vi "test_F9P_fgv-ver.vi"() -> ()   [LabVIEW 2019] (continued)
27,182,,07,09,201,18,1*72\r\n$GBGSV,4,2,13,08,65,355,33,09,07,194,,10,16,222,18,11,38,142,27,1*7C\r\n$GBGSV,4,3,13,13,50,314,20,14,77,038,37,28,58,310,28,33,72,237,41,1*73\r\n$GBGSV,4,4,13,34,13,141,,1*45\r\n$GBGSV,4,1,13,04,35,133,,05,09,257,,06,27,182,,07,09,201,,3*79\r\n$GBGSV,4,2,13,08,65,355,33,09,07,194,,10,16,222,19,11,38,142,26,3*7E\r\n$GBGSV,4,3,13,13,50,314,,14,77,038,38,28,58,310,,33,72,237,,3*73\r\n$GBGSV,4,4,13,34,13,141,,3*47\r\n$GNGLL,3723.61077,N,12656.95320,E,064222.00,A,A*7E\r\n$GNRMC,064223.00,A,3723.61113,N,12656.95407,E,2.484,70.88,250720,,,A,V*3C\r\n$GNVTG,70.88,T,,M,2.484,N,4.600,K,A*1C\r\n$GNGGA,064223.00,3723.61113,N,12656.95407,E,1,12,0.73,46.5,M,18.5,M,,*77\r\n$GNGSA,A,3,17,19,06,05,02,12,09,,,,,,1.16,0.73,0.90,1*0F\r\n$GNGSA,A,3,85,70,71,72,,,,,,,,,1.16,0.73,0.90,2*00\r\n$GNGSA,A,3,36,19,11,04,09,12,,,,,,,1.16,0.73,0.90,3*0B\r\n$GNGSA,A,3,28,14,13,11,33,08,10,,,,,,1.16,0.73,0.90,4*0B\r\n$GPGSV,4,1,13,02,65,334,31,04,08,037,26,05,48,261,35,06,58,076,40,1*6C\r\n$GPGSV,4,2,13,07,06,105,,09,38,057,43,12,18,263,24,13,08,191,,1*6A\r\n$GPGSV,4,3,13,17,19,158,25,19,37,161,34,25,11,294,18,29,07,323,,1*66\r\n$GPGSV,4,4,13,30,01,134,,1*52\r\n$GPGSV,4,1,13,02,65,334,,04,08,037,20,05,48,261,26,06,58,076,31,6*6B\r\n$GPGSV,4,2,13,07,06,105,,09,38,057,40,12,18,263,14,13,08,191,,6*6D\r\n$GPGSV,4,3,13,17,19,158,19,19,37,161,,25,11,294,,29,07,323,,6*60\r\n$GPGSV,4,4,13,30,01,134,,6*55\r\n$GLGSV,2,1,06,70,55,030,38,71,68,223,41,72,17,216,26,84,09,133,10,1*7B\r\n$GLGSV,2,2,06,85,63,111,34,86,51,337,,1*7D\r\n$GLGSV,2,1,06,70,55,030,,71,68,223,28,72,17,216,20,84,09,133,10,3*7B\r\n$GLGSV,2,2,06,85,63,111,25,86,51,337,,3*7F\r\n$GAGSV,3,1,09,02,04,287,10,04,68,085,41,09,44,196,30,11,78,037,38,7*74\r\n$GAGSV,3,2,09,12,32,114,28,18,55,286,40,19,17,042,27,25,01,241,,7*7A\r\n$GAGSV,3,3,09,36,34,314,23,7*4F\r\n$GAGSV,3,1,09,02,04,287,,04,68,085,31,09,44,196,28,11,78,037,31,2*77\r\n$GAGSV,3,2,09,12,32,114,25,18,55,286,43,19,17,042,25,25,01,241,,2*73\r\n$GAGSV,3,3,09,36,34,314,19,2*43\r\n$GBGSV,4,1,13,04,35,133,,05,09,257,,06,27,182,,07,09,201,19,1*73\r\n$GBGSV,4,2,13,08,65,355,39,09,07,194,,10,16,222,17,11,38,142,26,1*78\r\n$GBGSV,4,3,13,13,50,314,20,14,77,038,38,28,58,310,28,33,72,237,42,1*7F\r\n$GBGSV,4,4,13,34,13,141,,1*45\r\n$GBGSV,4,1,13,04,35,133,,05,09,257,,06,27,182,,07,09,201,,3*79\r\n$GBGSV,4,2,13,08,65,355,37,09,07,194,,10,16,222,20,11,38,142,30,3*77\r\n$GBGSV,4,3,13,13,50,314,,14,77,038,40,28,58,310,,33,72,237,,3*7C\r\n$GBGSV,4,4,13,34,13,141,,3*47\r\n$GNGLL,3723.61113,N,12656.95407,E,064223.00,A,A*7E\r\n$GNRMC,064224.00,A,3723.61154,N,12656.95489,E,2.441,65.71,250720,,,A,V*35\r\n$GNVTG,65.71,T,,M,2.441,N,4.520,K,A*16\r\n$GNGGA,064224.00,3723.61154,N,12656.95489,E,1,12,0.73,46.1,M,18.5,M,,*71\r\n$GNGSA,A,3,17,19,06,05,02,12,09,,,,,,1.16,0.73,0.90,1*0F\r\n$GNGSA,A,3,85,70,71,72,,,,,,,,,1.16,0.73,0.90,2*00\r\n$GNGSA,A,3,36,19,11,04,09,12,,,,,,,1.16,0.73,0.90,3*0B\r\n$GNGSA,A,3,28,14,13,11,33,08,10,,,,,,1.16,0.73,0.90,4*0B\r\n$GPGSV,4,1,13,02,65,334,26,04,08,037,32,05,48,261,35,06,58,076,42,1*6D\r\n$GPGSV,4,2,13,07,06,105,,09,38,057,44,12,18,263,23,13,08,191,,1*6A\r\n$GPGSV,4,3,13,17,19,158,26,19,37,161,31,25,11,294,18,29,07,323,,1*60\r\n$GPGSV,4,4,13,30,01,134,,1*52\r\n$GPGSV,4,1,13,02,65,334,,04,08,037,20,05,48,261,26,06,58,076,32,6*68\r\n$GPGSV,4,2,13,07,06,105,,09,38,057,39,12,18,263,15,13,08,191,,6*62\r\n$GPGSV,4,3,13,17,19,158,21,19,37,161,,25,11,294,,29,07,323,,6*6B\r\n$GPGSV,4,4,13,30,01,134,,6*55\r\n$GLGSV,2,1,06,70,55,030,36,71,68,223,42,72,17,216,35,84,09,133,10,1*74\r\n$GLGSV,2,2,06,85,63,111,25,86,51,337,,1*7D\r\n$GLGSV,2,1,06,70,55,030,,71,68,223,28,72,17,216,21,84,09,133,10,3*7A\r\n$GLGSV,2,2,06,85,63,111,24,86,51,337,,3*7E\r\n$GAGSV,3,1,09,02,04,287,09,04,68,085,37,09,44,196,29,11,78,037,36,7*7B\r\n$GAGSV,3,2,09,12,32,114,32,18,55,286,35,19,17,042,28,25,01,241,,7*7C\r\n$GAGSV,3,3,09,36,34,314,24,7*48\r\n$GAGSV,3,1,09,02,04,287,,04,68,085,35,09,44,196,27,11,78,037,32,2*7F\r\n$GAGSV,3,2,09,12,32,114,25,18,55,286,43,19,17,042,31,25,01,241,,2*76\r\n$GAGSV,3,3,09,36,34,314,19,2*43\r\n$GBGSV,4,1,13,04,35,133,,05,09,257,,06,27,182,,07,09,201,20,1*79\r\n$GBGSV,4,2,13,08,65,355,40,09,07,194,,10,16,222,16,11,38,142,27,1*76\r\n$GBGSV,4,3,13,13,50,314,19,14,77,038,42,28,58,310,26,33,72,237,33,1*70\r\n$GBGSV,4,4,13,34,13,141,,1*45\r\n$GBGSV,4,1,13,04,35,133,,05,09,257,,06,27,182,,07,09,201,,3*79\r\n$GBGSV,4,2,13,08,65,355,36,09,07,194,,10,16,222,20,11,38,142,29,3*7E\r\n$GBGSV,4,3,13,13,50,314,,14,77,038,37,28,58,310,,33,72,237,,3*7C\r\n$GBGSV,4,4,13,34,13,141,,3*47\r\n$GNGLL,3723.61154,N,12656.95489,E,064224.00,A,A*7C\r\n$GNRMC,064225.00,A,3723.61204,N,12656.95562,E,2.487,60.20,250720,,,A,V*3D\r\n$GNVTG,60.20,T,,M,2.487,N,4.606,K,A*1A\r\n$GNGGA,064225.00,3723.61204,N,12656.95562,E,1,12,0.76,45.7,M,18.5,M,,*72\r\n$GNGSA,A,3,17,19,06,05,02,12,09,,,,,,1.18,0.76,0.90,1*04\r\n$GNGSA,A,3,85,70,71,72,,,,,,,,,1.18,0.76,0.90,2*0B\r\n$GNGSA,A,3,36,19,11,04,09,12,,,,,,,1.18,0.76,0.90,3*00\r\n$GNGSA,A,3,28,14,13,11,33,08,10,,,,,,1.18,0.76,0.90,4*00\r\n$GPGSV,4,1,13,02,65,334,36,04,08,037,28,05,48,261,32,06,58,076,36,1*63\r\n$GPGSV,4,2,13,07,06,105,,09,38,057,43,12,18,263,25,13,08,191,,1*6B\r\n$GPGSV,4,3,13,17,19,158,26,19,37,161,26,25,11,294,17,29,07,323,,1*69\r\n$GPGSV,4,4,13,30,01,134,,1*52\r\n$GPGSV,4,1,13,02,65,334,,04,08,037,24,05,48,261,32,06,58,076,32,6*69\r\n$GPGSV,4,2,13,07,06,105,,09,38,057,39,12,18,263,15,13,08,191,,6*62\r\n$GPGSV,4,3,13,17,19,158,20,19,37,161,,25,11,294,,29,07,323,,6*6A\r\n$GPGSV,4,4,13,30,01,134,,6*55\r\n$GLGSV,2,1,06,70,55,030,40,71,68,223,37,72,17,216,30,84,09,133,07,1*74\r\n$GLGSV,2,2,06,85,63,111,34,86,51,337,,1*7D\r\n$GLGSV,2,1,06,70,55,030,,71,68,223,23,72,17,216,21,84,09,133,10,3*71\r\n$GLGSV,2,2,06,85,63,111,24,86,51,337,,3*7E\r\n$GAGSV,3,1,09,02,04,287,09,04,68,085,37,09,44,196,30,11,78,037,39,7*7C\r\n$GAGSV,3,2,09,12,32,114,25,18,55,286,31,19,17,042,26,25,01,241,,7*70\r\n$GAGSV,3,3,09,36,34,314,25,7*49\r\n$GAGSV,3,1,09,02,04,287,,04,68,085,30,09,44,196,29,11,78,037,35,2*73\r\n$GAGSV,3,2,09,12,32,114,30,18,55,286,36,19,17,042,32,25,01,241,,2*73\r\n$GAGSV,3,3,09,36,34,314,19,2*43\r\n$GBGSV,4,1,13,04,35,133,,05,09,257,,06,27,182,,07,09,201,22,1*7B\r\n$GBGSV,4,2,13,08,65,355,41,09,07,194,,10,16,222,15,11,38,142,32,1*70\r\n$GBGSV,4,3,13,13,50,314,18,14,77,038,44,28,58,310,26,33,72,237,39,1*7D\r\n$GBGSV,4,4,13,34,13,141,,1*45\r\n$GBGSV,4,1,13,04,35,133,,05,09,257,,06,27,182,,07,09,201,,3*79\r\n$GBGSV,4,2,13,08,65,355,37,09,07,194,,10,16,222,20,11,38,142,28,3*7E\r\n$GBGSV,4,3,13,13,50,314,,14,77,038,38,28,58,310,,33,72,237,,3*73\r\n$GBGSV,4,4,13,34,13,141,,3*47\r\n$GNGLL,3723.61204,N,12656.95562,E,064225.00,A,A*7F\r\n$GNRMC,064226.00,A,3723.61239,N,12656.95636,E,2.337,64.01,250720,,,A,V*39\r\n$GNVTG,64.01,T,,M,2.337,N,4.329,K,A*19\r\n$GNGGA,064226.00,3723.61239,N,12656.95636,E,1,12,0.68,45.0,M,18.5,M,,*75\r\n$GNGSA,A,3,17,19,06,05,02,12,09,,,,,,1.13,0.68,0.90,1*00\r\n$GNGSA,A,3,85,70,71,72,,,,,,,,,1.13,0.68,0.90,2*0F\r\n$GNGSA,A,3,36,19,11,04,09,12,,,,,,,1.13,0.68,0.90,3*04\r\n$GNGSA,A,3,28,14,13,11,33,08,10,,,,,,1.13,0.68,0.90,4*04\r\n$GPGSV,4,1,13,02,65,334,42,04,08,037,36,05,48,261,36,06,58,076,35,1*68\r\n$GPGSV,4,2,13,07,06,105,,09,38,057,44,12,18,263,26,13,08,191,,1*6F\r\n$GPGSV,4,3,13,17,19,158,25,19,37,161,27,25,11,294,15,29,07,323,,1*69\r\n$GPGSV,4,4,13,30,01,134,,1*52\r\n$GPGSV,4,1,13,02,65,334,,04,08,037,25,05,48,261,35,06,58,076,26,6*6A\r\n$GPGSV,4,2,13,07,06,105,,09,38,057,41,12,18,263,15,13,08,191,,6*6D\r\n$GPGSV,4,3,13,17,19,158,19,19,37,161,,25,11,294,,29,07,323,,6*60\r\n$GPGSV,4,4,13,30,01,134,,6*55\r\n$GLGSV,2,1,06,70,55,030,35,71,68,223,41,72,17,216,26,84,09,133,08,1*7F\r\n$GLGSV,2,2,06,85,63,111,33,86,51,337,,1*7A\r\n$GLGSV,2,1,06,70,55,030,,71,68,223,32,72,17,216,20,84,09,133,11,3*71\r\n$GLGSV,2,2,06,85,63,111,24,86,51,337,,3*7E\r\n$GAGSV,3,1,09,02,04,287,10,04,68,085,35,09,44,196,31,11,78,037,40,7*79\r\n$GAGSV,3,2,09,12,32,114,25,18,55,284,32,19,17,042,31,25,01,241,,7*77\r\n$GAGSV,3,3,09,36,34,314,26,7*4A\r\n$GAGSV,3,1,09,02,04,287,,04,68,085,34,09,44,196,29,11,78,037,34,2*76\r\n$GAGSV,3,2,09,12,32,114,28,18,55,284,38,19,17,042,39,25,01,241,,2*7D\r\n$GAGSV,3,3,09,36,34,314,21,2*48\r\n$GBGSV,4,1,13,04,35,133,,05,09,257,,06,27,182,,07,09,201,23,1*7A\r\n$GBGSV,4,2,13,08,65,355,42,09,07,194,,10,16,222,18,11,38,142,25,1*78\r\n$GBGSV,4,3,13,13,50,314,19,14,77,038,41,28,58,310,26,33,72,237,40,1*77\r\n$GBGSV,4,4,13,34,13,141,,1*45\r\n$GBGSV,4,1,13,04,35,133,,05,09,257,,06,27,182,,07,09,201,,3*79\r\n$GBGSV,4,2,13,08,65,355,34,09,07,194,,10,16,222,20,11,38,142,28,3*7D\r\n$GBGSV,4,3,13,13,50,314,,14,77,038,38,28,58,310,,33,72,237,,3*73\r\n$GBGSV,4,4,13,34,13,141,,3*47\r\n$GNGLL,3723.61239,N,12656.95636,E,064226.00,A,A*70\r\n$GNRMC,064227.00,A,3723.61269,N,12656.95722,E,2.639,65.95,250720,,,A,V*3E\r\n$GNVTG,65.95,T,,M,2.639,N,4.887,K,A*11\r\n$GNGGA,064227.00,3723.61269,N,12656.95722,E,1,12,0.66,44.4,M,18.5,M,,*7E\r\n$GNGSA,A,3,17,19,06,05,02,12,09,,,,,,1.11,0.66,0.89,1*04\r\n$GNGSA,A,3,85,70,71,72,,,,,,,,,1.11,0.66,0.89,2*0B\r\n$GNGSA,A,3,36,19,11,04,09,12,,,,,,,1.11,0.66,0.89,3*00\r\n$GNGSA,A,3,28,14,13,11,33,08,10,,,,,,1.11,0.66,0.89,4*00\r\n$GPGSV,4,1,13,02,65,334,42,04,08,037,32,05,48,261,29,06,58,076,36,1*61\r\n$GPGSV,4,2,13,07,06,105,,09,38,057,49,12,18,263,24,13,08,191,,1*60\r\n$GPGSV,4,3,13,17,19,158,24,19,37,161,26,25,11,294,17,29,07,323,,1*6B\r\n$GPGSV,4,4,13,30,01,134,,1*52\r\n$GPGSV,4,1,13,02,65,334,,04,08,037,25,05,48,261,28,06,58,076,35,6*64\r\n$GPGSV,4,2,13,07,06,105,,09,38,057,39,12,18,263,15,13,08,191,,6*62\r\n$GPGSV,4,3,13,17,19,158,19,19,37,161,,25,11,294,,29,07,323,,6*60\r\n$GPGSV,4,4,13,30,01,134,,6*55\r\n$GLGSV,2,1,06,70,55,030,33,71,68,223,42,72,17,216,26,84,09,133,11,1*72\r\n$GLGSV,2,2,06,85,63,111,31,86,51,337,,1*78\r\n$GLGSV,2,1,06,70,55,030,,71,68,223,26,72,17,216,18,84,09,133,11,3*7F\r\n$GLGSV,2,2,06,85,63,111,26,86,51,337,,3*7C\r\n$GAGSV,3,1,09,02,04,287,10,04,68,085,35,09,44,196,30,11,78,037,39,7*76\r\n$GAGSV,3,2,09,12,32,114,32,18,55,284,39,19,17,042,39,25,01,241,,7*72\r\n$GAGSV,3,3,09,36,34,314,26,7*4A\r\n$GAGSV,3,1,09,02,04,287,,04,68,085,30,09,44,196,21,11,78,037,30,2*7E\r\n$GAGSV,3,2,09,12,32,114,28,18,55,284,44,19,17,042,39,25,01,241,,2*76\r\n$GAGSV,3,3,09,36,34,314,21,2*48\r\n$GBGSV,4,1,13,04,35,133,,05,09,257,,06,27,182,,07,09,201,22,1*7B\r\n$GBGSV,4,2,13,08,65,355,39,09,07,194,,10,16,222,17,11,38,142,26,1*78\r\n$GBGSV,4,3,13,13,50,314,20,14,77,038,44,28,58,310,24,33,72,237,40,1*7A\r\n$GBGSV,4,4,13,34,13,141,,1*45\r\n$GBGSV,4,1,13,04,35,133,,05,09,257,,06,27,182,,07,09,201,,3*79\r\n$GBGSV,4,2,13,08,65,355,36,09,07,194,,10,16,222,20,11,38,142,22,3*75\r\n$GBGSV,4,3,13,13,50,314,,14,77,038,36,28,58,310,,33,72,237,,3*7D\r\n$GBGSV,4,4,13,34,13,141,,3*47\r\n$GNGLL,3723.61269,N,12656.95722,E,064227.00,A,A*70\r\n$GNRMC,064228.00,A,3723.61290,N,12656.95811,E,2.772,74.12,250720,,,A,V*39\r\n$GNVTG,74.12,T,,M,2.772,N,5.133,K,A*17\r\n$GNGGA,064228.00,3723.61290,N,12656.95811,E,1,12,0.68,43.8,M,18.5,M,,*7D\r\n$GNGSA,A,3,17,19,06,05,02,12,09,,,,,,1.13,0.68,0.90,1*00\r\n$GNGSA,A,3,85,70,71,72,,,,,,,,,1.13,0.68,0.90,2*0F\r\n$GNGSA,A,3,36,19,11,04,09,12,,,,,,,1.13,0.68,0.90,3*04\r\n$GNGSA,A,3,28,14,13,11,33,08,10,,,,,,1.13,0.68,0.90,4*04\r\n$GPGSV,4,1,13,02,65,334,42,04,08,037,36,05,48,261,29,06,58,076,39,1*6A\r\n$GPGSV,4,2,13,07,06,105,,09,38,057,45,12,18,263,22,13,08,191,,1*6A\r\n$GPGSV,4,3,13,17,19,158,23,19,37,161,27,25,11,294,17,29,07,323,,1*6D\r\n$GPGSV,4,4,13,30,01,134,,1*52\r\n$GPGSV,4,1,13,02,65,334,,04,08,037,25,05,48,261,33,06,58,076,31,6*6A\r\n$GPGSV,4,2,13,07,06,105,,09,38,057,43,12,18,263,16,13,08,191,,6*6C\r\n$GPGSV,4,3,13,17,19,158,18,19,37,161,,25,11,294,,29,07,323,,6*61\r\n$GPGSV,4,4,13,30,01,134,,6*55\r\n$GLGSV,2,1,06,70,55,030,29,71,68,223,32,72,17,216,26,84,09,133,08,1*76\r\n$GLGSV,2,2,06,85,63,111,25,86,51,337,,1*7D\r\n$GLGSV,2,1,06,70,55,030,,71,68,223,27,72,17,216,18,84,09,133,10,3*7F\r\n$GLGSV,2,2,06,85,63,111,24,86,51,337,,3*7E\r\n$GAGSV,3,1,09,02,04,287,07,04,68,085,35,09,44,196,29,11,78,037,35,7*74\r\n$GAGSV,3,2,09,12,32,114,30,18,55,284,34,19,17,042,36,25,01,241,,7*72\r\n$GAGSV,3,3,09,36,34,314,25,7*49\r\n$GAGSV,3,1,09,02,04,287,,04,68,085,29,09,44,196,23,11,78,037,33,2*77\r\n$GAGSV,3,2,09,12,32,114,22,18,55,284,41,19,17,042,38,25,01,241,,2*78\r\n$GAGSV,3,3,09,36,34,314,21,2*48\r\n$GBGSV,4,1,13,04,35,133,,05,09,257,,06,27,182,,07,09,201,22,1*7B\r\n$GBGSV,4,2,13,08,65,355,38,09,07,194,,10,16,222,17,11,38,142,27,1*78\r\n$GBGSV,4,3,13,13,50,314,19,14,77,038,38,28,58,310,25,33,72,237,40,1*7A\r\n$GBGSV,4,4,13,34,13,141,,1*45\r\n$GBGSV,4,1,13,04,35,133,,05,09,257,,06,27,182,,07,09,201,,3*79\r\n$GBGSV,4,2,13,08,65,355,38,09,07,194,,10,16,222,19,11,38,142,33,3*71\r\n$GBGSV,4,3,13,13,50,314,,14,77,038,39,28,58,310,,33,72,237,,3*72\r\n$GBGSV,4,4,13,34,13,141,,3*47\r\n$GNGLL,3723.61290,N,12656.95811,E,064228.00,A,A*76\r\n$GNRMC,064229.00,A,3723.61320,N,12656.95903,E,2.398,72.65,250720,,,A,V*36\r\n$GNVTG,72.65,T,,M,2.398,N,4.441,K,A*10\r\n$GNGGA,064229.00,3723.61320,N,12656.95903,E,1,12,0.70,43.6,M,18.5,M,,*73\r\n$GNGSA,A,3,17,19,06,05,02,12,09,,,,,,1.14,0.70,0.90,1*0E\r\n$GNGSA,A,3,85,70,71,72,,,,,,,,,1.14,0.70,0.90,2*01\r\n$GNGSA,A,3,36,19,11,04,09,12,,,,,,,1.14,0.70,0.90,3*0A\r\n$GNGSA,A,3,28,14,13,11,33,08,10,,,,,,1.14,0.70,0.90,4*0A\r\n$GPGSV,4,1,13,02,65,334,42,04,08,037,35,05,48,261,33,06,58,076,37,1*6C\r\n$GPGSV,4,2,13,07,06,105,,09,38,057,43,12,18,263,24,13,08,191,,1*6A\r\n$GPGSV,4,3,13,17,19,158,24,19,37,161,26,25,11,294,16,29,07,323,,1*6A\r\n$GPGSV,4,4,13,30,01,134,,1*52\r\n$GPGSV,4,1,13,02,65,334,,04,08,037,25,05,48,261,32,06,58,076,31,6*6B\r\n$GPGSV,4,2,13,07,06,105,,09,38,057,40,12,18,263,15,13,08,191,,6*6C\r\n$GPGSV,4,3,13,17,19,158,17,19,37,161,,25,11,294,,29,07,323,,6*6E\r\n$GPGSV,4,4,13,30,01,134,,6*55\r\n$GLGSV,2,1,06,70,55,030,35,71,68,223,40,72,17,216,26,84,09,133,08,1*7E\r\n$GLGSV,2,2,06,85,63,111,34,86,51,337,,1*7D\r\n$GLGSV,2,1,06,70,55,030,,71,68,223,26,72,17,216,20,84,09,133,10,3*75\r\n$GLGSV,2,2,06,85,63,111,30,86,51,337,,3*7B\r\n$GAGSV,3,1,09,02,04,287,09,04,68,085,37,09,44,196,30,11,78,037,37,7*72\r\n$GAGSV,3,2,09,12,32,114,25,18,55,284,29,19,17,042,29,25,01,241,,7*74\r\n$GAGSV,3,3,09,36,34,314,24,7*48\r\n$GAGSV,3,1,09,02,04,287,,04,68,085,33,09,44,196,24,11,78,037,32,2*7A\r\n$GAGSV,3,2,09,12,32,114,24,18,55,284,41,19,17,042,37,25,01,241,,2*71\r\n$GAGSV,3,3,09,36,34,314,20,2*49\r\n$GBGSV,4,1,13,04,35,133,,05,09,257,,06,27,182,,07,09,201,21,1*78\r\n$GBGSV,4,2,13,08,65,355,38,09,07,194,,10,16,222,17,11,38,142,31,1*7F\r\n$GBGSV,4,3,13,13,50,314,20,14,77,038,42,28,58,310,26,33,72,237,42,1*7C\r\n$GBGSV,4,4,13,34,13,141,,1*45\r\n$GBGSV,4,1,13,04,35,133,,05,09,257,,06,27,182,,07,09,201,,3*79\r\n$GBGSV,4,2,13,08,65,355,29,09,07,194,,10,16,222,20,11,38,142,33,3*7B\r\n$GBGSV,4,3,13,13,50,314,,14,77,038,37,28,58,310,,33,72,237,,3*7C\r\n$GBGSV,4,4,13,34,13,141,,3*47\r\n$GNGLL,3723.61320,N,12656.95903,E,064229.00,A,A*7F\r\n$GNRMC,064230.00,A,3723.61332,N,12656.95977,E,1.999,77.80,250720,,,A,V*38\r\n$GNVTG,77.80,T,,M,1.999,N,3.702,K,A*15\r\n$GNGGA,064230.00,3723.61332,N,12656.95977,E,1,12,0.70,43.2,M,18.5,M,,*7F\r\n$GNGSA,A,3,17,19,06,05,02,12,09,,,,,,1.14,0.70,0.90,1*0E\r\n$GNGSA,A,3,85,70,71,72,,,,,,,,,1.14,0.70,0.90,2*01\r\n$GNGSA,A,3,36,19,11,04,09,12,,,,,,,1.14,0.70,0.90,3*0A\r\n$GNGSA,A,3,28,14,13,11,33,08,10,,,,,,1.14,0.70,0.90,4*0A\r\n$GPGSV,4,1,13,02,65,334,47,04,08,037,33,05,48,261,37,06,58,076,41,1*6A\r\n$GPGSV,4,2,13,07,06,105,,09,38,057,40,12,18,263,23,13,08,191,,1*6E\r\n$GPGSV,4,3,13,17,19,158,24,19,37,161,27,25,11,294,17,29,07,323,,1*6A\r\n$GPGSV,4,4,13,30,01,134,,1*52\r\n$GPGSV,4,1,13,02,65,334,,04,08,037,25,05,48,261,26,06,58,076,28,6*66\r\n$GPGSV,4,2,13,07,06,105,,09,38,057,37,12,18,263,15,13,08,191,,6*6C\r\n$GPGSV,4,3,13,17,19,158,16,19,37,161,,25,11,294,,29,07,323,,6*6F\r\n$GPGSV,4,4,13,30,01,134,,6*55\r\n$GLGSV,2,1,06,70,55,030,32,71,68,223,37,72,17,216,27,84,09,133,09,1*79\r\n$GLGSV,2,2,06,85,63,111,29,86,51,337,,1*71\r\n$GLGSV,2,1,06,70,55,030,,71,68,223,26,72,17,216,19,84,09,133,10,3*7F\r\n$GLGSV,2,2,06,85,63,111,24,86,51,337,,3*7E\r\n$GAGSV,3,1,09,02,04,287,09,04,68,085,40,09,44,196,30,11,78,037,34,7*71\r\n$GAGSV,3,2,09,12,32,114,29,18,55,284,28,19,17,042,33,25,01,241,,7*72\r\n$GAGSV,3,3,09,36,34,314,24,7*48\r\n$GAGSV,3,1,09,02,04,287,,04,68,085,35,09,44,196,31,11,78,037,31,2*7B\r\n$GAGSV,3,2,09,12,32,114,24,18,55,284,38,19,17,042,34,25,01,241,,2*7C\r\n$GAGSV,3,3,09,36,34,314,18,2*42\r\n$GBGSV,4,1,13,04,35,133,,05,09,257,,06,27,182,,07,09,201,20,1*79\r\n$GBGSV,4,2,13,08,65,355,41,09,07,194,,10,16,222,17,11,38,142,26,1*77\r\n$GBGSV,4,3,13,13,50,314,22,14,77,038,40,28,58,310,26,33,72,237,40,1*7E\r\n$GBGSV,4,4,13,34,13,141,,1*45\r\n$GBGSV,4,1,13,04,35,133,,05,09,257,,06,27,182,,07,09,201,,3*79\r\n$GBGSV,4,2,13,08,65,355,36,09,07,194,,10,16,222,20,11,38,142,33,3*75\r\n$GBGSV,4,3,13,13,50,314,17,14,77,038,39,28,58,310,,33,72,237,,3*74\r\n$GBGSV,4,4,13,34,13,141,,3*47\r\n$GNGLL,3723.61332,N,12656.95977,E,064230.00,A,A*77\r\n$GNRMC,064231.00,A,3723.61346,N,12656.96053,E,2.248,78.36,250720,,,A,V*30\r\n$GNVTG,78.36,T,,M,2.248,N,4.164,K,A*12\r\n$GNGGA,064231.00,3723.61346,N,12656.96053,E,1,12,0.73,43.0,M,18.5,M,,*70\r\n$GNGSA,A,3,17,19,06,05,02,12,09,,,,,,1.18,0.73,0.92,1*03\r\n$GNGSA,A,3,85,70,71,72,,,,,,,,,1.18,0.73,0.92,2*0C\r\n$GNGSA,A,3,36,19,11,04,09,12,,,,,,,1.18,0.73,0.92,3*07\r\n$GNGSA,A,3,28,14,13,11,33,08,10,,,,,,1.18,0.73,0.92,4*07\r\n$GPGSV,4,1,13,02,65,334,45,04,08,037,35,05,48,261,31,06,58,076,42,1*6B\r\n$GPGSV,4,2,13,07,06,105,,09,38,057,42,12,18,263,23,13,08,191,,1*6C\r\n$GPGSV,4,3,13,17,19,158,31,19,37,161,27,25,11,294,16,29,07,323,,1*6F\r\n$GPGSV,4,4,13,30,01,134,,1*52\r\n$GPGSV,4,1,13,02,65,334,,04,08,037,32,05,48,261,33,06,58,076,33,6*6E\r\n$GPGSV,4,2,13,07,06,105,,09,38,057,37,12,18,263,16,13,08,191,,6*6F\r\n$GPGSV,4,3,13,17,19,158,19,19,37,161,,25,11,294,,29,07,323,,6*60\r\n$GPGSV,4,4,13,30,01,134,,6*55\r\n$GLGSV,2,1,06,70,55,030,35,71,68,223,30,72,17,216,27,84,09,133,06,1*76\r\n$GLGSV,2,2,06,85,63,111,29,86,51,337,,1*71\r\n$GLGSV,2,1,06,70,55,030,,71,68,223,27,72,17,216,20,84,09,133,09,3*7C\r\n$GLGSV,2,2,06,85,63,111,24,86,51,337,,3*7E\r\n$GAGSV,3,1,09,02,04,287,11,04,68,085,37,09,44,196,29,11,78,037,38,7*7C\r\n$GAGSV,3,2,09,12,32,114,29,18,55,284,33,19,17,042,40,25,01,241,,7*7C\r\n$GAGSV,3,3,09,36,34,314,25,7*49\r\n$GAGSV,3,1,09,02,04,287,,04,68,085,33,09,44,196,29,11,78,037,31,2*74\r\n$GAGSV,3,2,09,12,32,114,24,18,55,284,39,19,17,042,34,25,01,241,,2*7D\r\n$GAGSV,3,3,09,36,34,314,20,2*49\r\n$GBGSV,4,1,13,04,35,133,,05,09,257,,06,27,182,,07,09,201,20,1*79\r\n$GBGSV,4,2,13,08,65,355,40,09,07,194,,10,16,222,16,11,38,142,29,1*78\r\n$GBGSV,4,3,13,13,50,314,22,14,77,038,41,28,58,310,26,33,72,237,37,1*7F\r\n$GBGSV,4,4,13,34,13,141,,1*45\r\n$GBGSV,4,1,13,04,35,133,,05,09,257,,06,27,182,,07,09,201,,3*79\r\n$GBGSV,4,2,13,08,65,355,36,09,07,194,,10,16,222,19,11,38,142,32,3*7E\r\n$GBGSV,4,3,13,13,50,314,,14,77,038,36,28,58,310,,33,72,237,,3*7D\r\n$GBGSV,4,4,13,34,13,141,,3*47\r\n$GNGLL,3723.61346,N,12656.96053,E,064231.00,A,A*79\r\n$GNRMC,064232.00,A,3723.61378,N,12656.96129,E,2.262,75.15,250720,,,A,V*36\r\n$GNVTG,75.15,T,,M,2.262,N,4.189,K,A*15\r\n$GNGGA,064232.00,3723.61378,N,12656.96129,E,1,12,0.70,43.0,M,18.5,M,,*71\r\n$GNGSA,A,3,17,19,06,05,02,12,09,,,,,,1.14,0.70,0.90,1*0E\r\n$GNGSA,A,3,85,70,71,72,,,,,,,,,1.14,0.70,0.90,2*01\r\n$GNGSA,A,3,36,19,11,04,09,12,,,,,,,1.14,0.70,0.90,3*0A\r\n$GNGSA,A,3,28,14,13,11,33,08,10,,,,,,1.14,0.70,0.90,4*0A\r\n$GPGSV,4,1,13,02,65,334,45,04,08,037,32,05,48,261,36,06,58,076,43,1*6A\r\n$GPGSV,4,2,13,07,06,105,,09,38,057,33,12,18,263,26,13,08,191,22,1*6F\r\n$GPGSV,4,3,13,17,19,158,25,19,37,161,30,25,11,294,18,29,07,323,,1*62\r\n$GPGSV,4,4,13,30,01,134,,1*52\r\n$GPGSV,4,1,13,02,65,334,,04,08,037,27,05,48,261,35,06,58,076,36,6*69\r\n$GPGSV,4,2,13,07,06,105,,09,38,057,41,12,18,263,16,13,08,191,,6*6E\r\n$GPGSV,4,3,13,17,19,158,20,19,37,161,,25,11,294,,29,07,323,,6*6A\r\n$GPGSV,4,4,13,30,01,134,,6*55\r\n$GLGSV,2,1,06,70,55,030,32,71,68,223,30,72,17,216,27,84,09,133,
